vi "Network.vi"() -> ()   [LabVIEW 2012, in "Phidget Common.lvlib"]
uses:
  <instrlib>/Phidgets/Phidget Common/Phidget Common.lvlib
  <instrlib>/Phidgets/Phidget Accelerometer/Public/AccelerometerStart.vi
  <instrlib>/Phidgets/Phidget Accelerometer/Public/AccelerometerClose.vi
  <instrlib>/Phidgets/Phidget Accelerometer/Phidget Accelerometer.lvlib
panel:
  out "Acceleration":dbl[](array[numeric])
  out "error out":errorcluster
  in  "Device Info":T1={"Serial Number"=-1, "Channel"=0, "Port"=0}
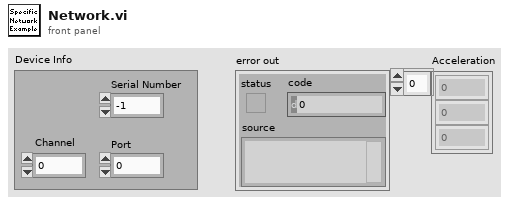
[diagram p1: front panel]
types:
  T1 = cluster{"Serial Number":i32, "Channel":i32, "Port":i32}
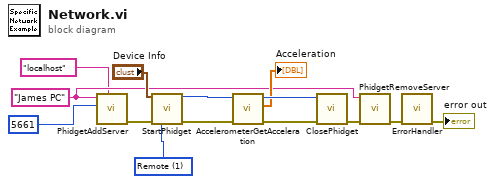
[diagram p0: block diagram]
diagram:
  w3 = "James PC" ("Name")
  w14 = u16 1 items=["No Preference", "Remote", "Local"] ("Connection")
  n1 = call <instrlib>:"PhidgetAddServer.vi"("Host"="localhost", "Port"=5661, "Name"=w3) -> ("error out"=w5:errorcluster)  [unwired: 8 in]
  n2 = call-poly <instrlib>:"StartPhidget.vi"("Device Info"="Device Info", "error in (no error)"=w5, "Connection"=w14) -> ("Phidget ID"=w11:u64, "error out"=w12:errorcluster)  [unwired: 9 in, 2 out]
  n3 = call <instrlib>:"AccelerometerGetAcceleration.vi"("error in (no error)"=w12, "Device In"=w11) -> ("error out"=w10:errorcluster, "Acceleration"=→"Acceleration":dbl[], "Device Out"=w9:u64)  [unwired: 6 in]
  n4 = call-poly <instrlib>:"ClosePhidget.vi"("error in"=w10, "Device In"=w9) -> ("error out"=w7:errorcluster)  [unwired: 9 in]
  n5 = call <instrlib>:"PhidgetRemoveServer.vi"("error in"=w7, "name"=w3) -> ("error out"=w6:errorcluster)  [unwired: 9 in]
  n6 = call <instrlib>:"ErrorHandler.vi"("error in"=w6) -> ("error out"=→"error out":errorcluster)  [unwired: 9 in, 1 out]
